vi "write module async property.vi"(7 "Module ID":string, 8 "error in":errorcluster, 10 "async?":bool, 11 "Standard Engine Repo Data in":refnum<class "Standard Engine Configuration.lvclass">) -> (0 "error out":errorcluster, 3 "Standard Engine Repo Data out":refnum<class "Standard Engine Configuration.lvclass">)   [LabVIEW 2013, in "Standard Engine Configuration.lvclass"]
uses:
  Standard Engine Configuration.lvclass
  Standard Engine Configuration.lvclass/Standard Engine Configuration.ctl
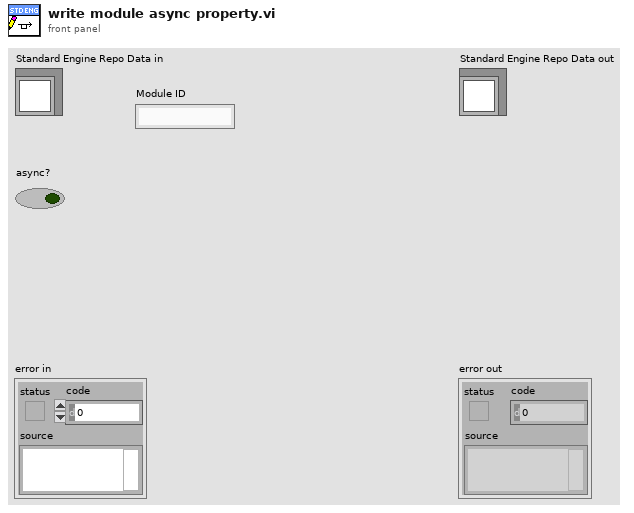
[diagram p1: front panel]
types:
  T1 = typedef "Standard Engine Configuration.lvclass/Module Specific Configuration.ctl" = cluster{"Module ID":string, "Module Decimation":T2, "Module Error Configuration":T3, "execution order priority":i32, "async?":bool, "report error?":bool, "error tag":string}
  T2 = typedef "Standard Engine Configuration.lvclass/Module Decimation.ctl" = cluster{"Decimation":u16, "Offset":u16}
  T3 = typedef "Standard Engine Configuration.lvclass/Module Error Configuration.ctl" = cluster{"Module Error Configuration":T4[]}
  T4 = typedef "Standard Engine Configuration.lvclass/Error Actions By Category.ctl" = cluster{"error classification":T5, "Error Actions":T6[]}
  T5 = typedef "TBM module execution interface.lvclass/error classification.ctl" = enum16{"unknown", "none", "trivial", "recoverable", "critical"}
  T6 = typedef "Standard Engine Configuration.lvclass/Error Actions.ctl" = enum16{"Clear", "Notify", "Stop Component", "Stop Engine", "Safe State", "Attempt Recovery"}
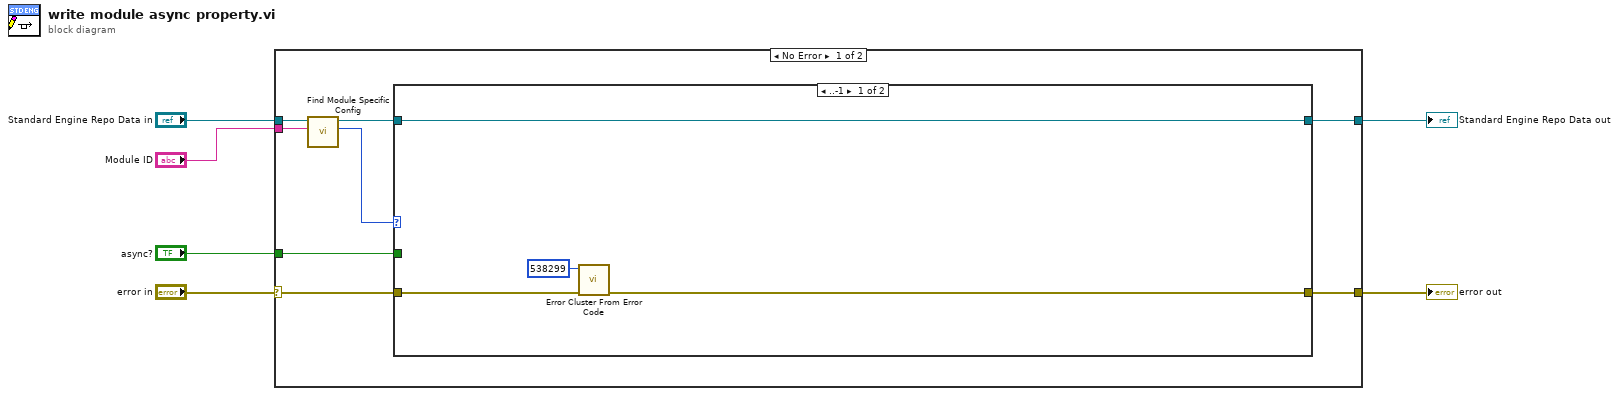
[diagram p0: block diagram]
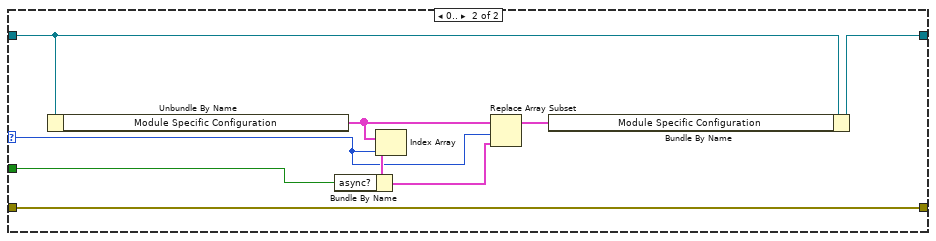
[diagram p2: hidden frame]
diagram:
  n1 = case shown="No Error" "error in" {
    selector: "error in" -> [w10 w29]
    tunnel: "Standard Engine Repo Data in" -> [w14 w28]
    tunnel: "Module ID" -> [w13 _]
    tunnel: [w8 w28] -> w2
    tunnel: [w9 w29] -> w3
    tunnel: "async?" -> [w7 _]
    frame No Error {
      n2 = call "Find Module Specific Config.vi"("Module ID"=w13, "Standard Engine Repo Data in"=w14) -> ("Index"=w11:i32, "Standard Engine Repo Data out"=w12:refnum<class "Standard Engine Configuration.lvclass">)  [unwired: 8 in]
      n3 = case shown="..-1" w11 {
        selector: w11 -> [_ w25]
        tunnel: w12 -> [w17 w22]
        tunnel: w10 -> [w18 w27]
        tunnel: [w16 w27] -> w9
        tunnel: [w17 w20] -> w8
        tunnel: w7 -> [_ w19]
        frame ..-1 {
          n4 = call <vilib>:"Error Cluster From Error Code.vi"("error in (no error)"=w18, "error code (0)"=538299) -> ("error out"=w16:errorcluster)  [unwired: 7 in]
        }
        frame 0.. {
          n5 = Unbundle By Name(w22) -> ("Module Specific Configuration"=w24:T1[])
          n6 = Index Array(array=w24, index=w25) -> (element=w26:T1)
          n7 = Bundle By Name(cluster=w26, "async?"=w19) -> (w23:T1)
          n8 = Replace Array Subset(array=w24, new element=w23, index=w25) -> (w21:T1[])
          n9 = Bundle By Name(cluster=w22, "Module Specific Configuration"=w21) -> (w20:refnum<class "Standard Engine Configuration.lvclass">)
        }
      }
    }
    frame Error {
    }
  }
  "error out" <- w3
  "Standard Engine Repo Data out" <- w2
